vi "Send datagram over TCP.vi"(7 "Data":i32[](array[numeric]), 8 "error in (no error)":errorcluster, 11 "connection ID":refnum<k5>) -> (0 "error out":errorcluster)   [LabVIEW 2015]
panel:
  out "iterrations":i32
  out "size(s)":i32
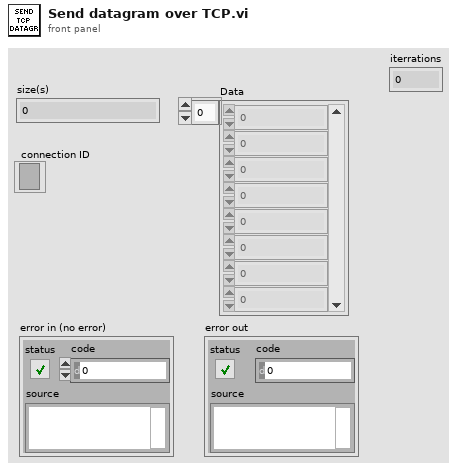
[diagram p1: front panel]
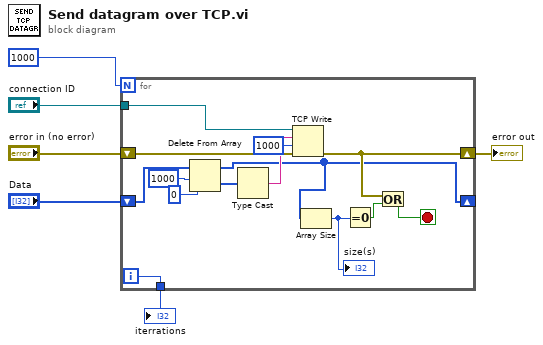
[diagram p0: block diagram]
diagram:
  n1 = for {
    N: 1000 -> [_]
    shift-right: [w12] -> w6
    shift-left: "error in (no error)" -> [w20]
    shift-right: [w8] -> _
    shift-left: "Data" -> [w18]
    tunnel: "connection ID" -> [w15]
    tunnel: [w13] -> w1
    i -> [w13]
    stop <- w10 stop-if-true
    n2 = Delete From Array(array=w18, length=1000, index=0) -> (deleted portion=w16:i32[], array with subset deleted=w8:i32[])
    n3 = Type Cast(x=w16) -> (*(type *) &x=w14:string)  [unwired: 1 in]
    n4 = TCP Write(connection ID=w15, data in=w14, error in (no error)=w20, 9:1000 ("timeout ms (25000)")) -> (error out=w12:errorcluster)  [unwired: 2 out]
    n5 = Array Size(array=w8) -> (size(s)=w19:i32)
    "size(s)" <- w19
    n6 = Equal To 0?(x=w19) -> (x = 0?=w11:bool)
    n7 = Or(x=w12, y=w11) -> (x .or. y?=w10:bool)
  }
  "error out" <- w6
  "iterrations" <- w1
